vi "FTW-Time-Remaining.vi"(0 "Total Work Units":i64, 5 "Work Units Complete":i64, 7 "Initial Timestamp":u32, 9 "Current Timestamp":u32, 11 "Window Size (for smoothing)":i32=15) -> (4 "Percent Done (0.0-100.0%)":dbl, 6 "Time Elapsed (msec)":u32, 8 "Estimated Time Remaining (msec)":u32, 10 "Current Rate (Units of Work per sec)":dbl, 15 "Settled?":bool)   [LabVIEW 2014]
panel:
  # "Inputs"
  # "Outputs"
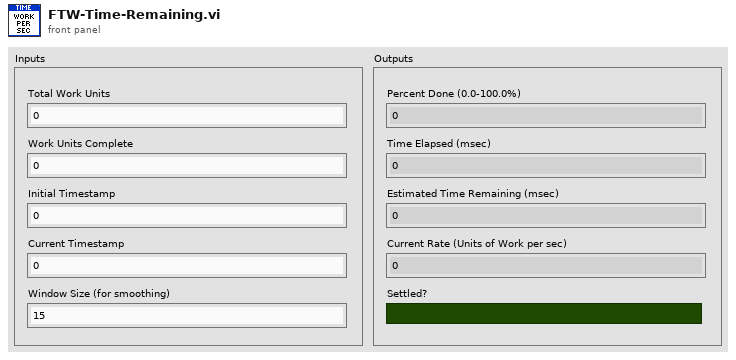
[diagram p1: front panel]
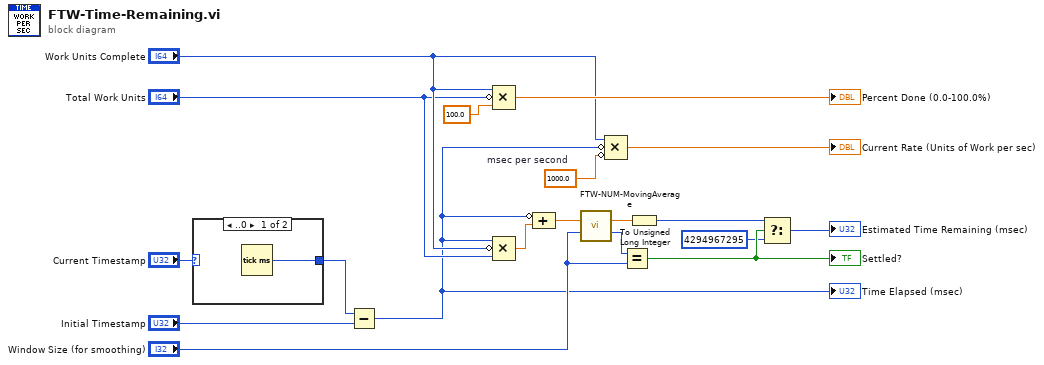
[diagram p0: block diagram]
diagram:
  w2 = 1000.0  # msec per second
  n1 = case shown="..0" "Current Timestamp" {
    selector: "Current Timestamp" -> [_ w21]
    tunnel: [w20 w21] -> w3
    frame ..0 {
      n2 = Tick Count (ms)() -> (millisecond timer value=w20:u32)
    }
    frame Default {
    }
  }
  n3 = Subtract(x=w3, y="Initial Timestamp") -> (x-y=w1:u32)
  "Time Elapsed (msec)" <- w1
  n4 = Compound Arithmetic op=MULTIPLY("Work Units Complete", invert "Total Work Units", 100.0 ("value")) -> (→"Percent Done (0.0-100.0%)":dbl)
  n5 = Compound Arithmetic op=MULTIPLY(w1, invert "Work Units Complete", "Total Work Units") -> (w19:dbl)
  n6 = Compound Arithmetic op=ADD(invert w1, w19) -> (w12:dbl)
  n7 = call "FTW-NUM-MovingAverage.vi"("New Value"=w12, "Window Size"="Window Size (for smoothing)") -> ("Average Value"=w8:dbl, "Items in Window"=w11:i32)  [unwired: 11 in, 1 out]
  n8 = Compound Arithmetic op=MULTIPLY("Work Units Complete", invert w1, invert w2) -> (→"Current Rate (Units of Work per sec)":dbl)
  n9 = Equal?(x=w11, y="Window Size (for smoothing)") -> (x = y?=w9:bool)
  "Settled?" <- w9
  n10 = To Unsigned Long Integer(number=w8) -> (unsigned 32bit integer=w5:u32)
  n11 = Select(t=w5, s=w9, f=u32 4294967295) -> (s? t:f=→"Estimated Time Remaining (msec)":u32)
